vi "Result Combine.vi"(11 "content":u8) -> (3 "result":u32)   [LabVIEW 2017, in "HD44780 FPGA.lvlib"]
uses:
  HD44780 FPGA.lvlib
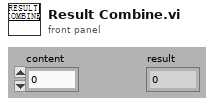
[diagram p1: front panel]
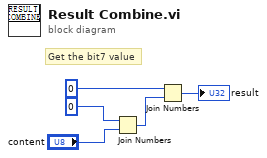
[diagram p0: block diagram]
diagram:
  # "Get the bit7 value"
  n1 = Join Numbers(hi=u8 0, lo="content") -> ((hi.lo)=w4:u16)
  n2 = Join Numbers(hi=u16 0, lo=w4) -> ((hi.lo)=→"result":u32)
